vi "GetFileCreationDate.vi"(6 "error in (no error)":errorcluster, 9 "File Path":path) -> (0 "error out":errorcluster, 3 "File Created Date (UTC)":timestamp)   [LabVIEW 2010, in "CAN Log Transfer and Convert.lvlib"]
uses:
  CAN Log Transfer and Convert.lvlib
  kernel32.dll
panel:
  in  "date time rec":T1
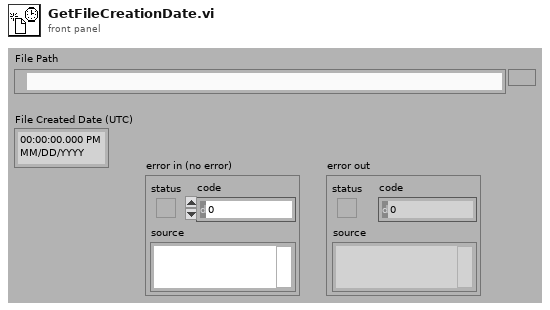
[diagram p1: front panel]
types:
  T1 = cluster{"fractional second":dbl, "second":i32, "minute":i32, "hour":i32, "day of month":i32, "month":i32, "year":i32, "day of week":i32, "day of year":i32, "DST":i32}
  T2 = cluster{"wYear":u16, "wMonth":u16, "wDayOfWeek":u16, "wDay":u16, "wHour":u16, "wMinute":u16, "wSeconds":u16, "wMilliseconds":u16}
  T3 = cluster{"dwFileAttributes":i32, "ftCreationTime":cluster{"dwLowDateTime":i32, "dwHighDateTime":i32}, "ftLastAccessTime":cluster{"dwLowDateTime":i32, "dwHighDateTime":i32}, "ftLastWrittenTime":cluster{"dwLowDateTime":i32, "dwHighDateTime":i32}, "nFileSizeHigh":i32, "nFileSizeLow":i32}
  T4 = cluster{"dwLowDateTime":i32, "dwHighDateTime":i32}
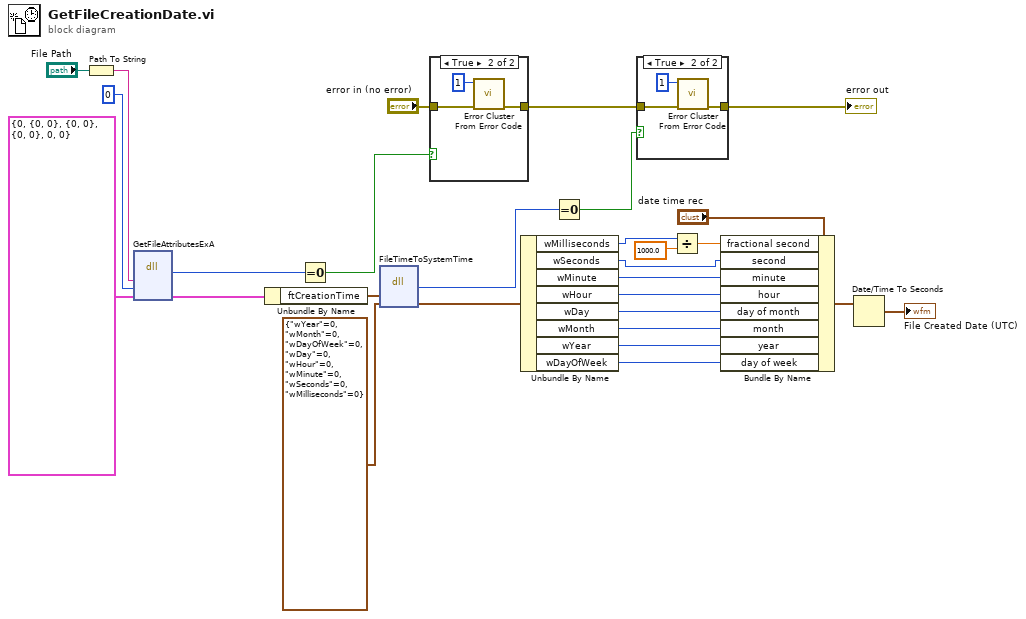
[diagram p0: block diagram]
diagram:
  n1 = Path To String(path="File Path") -> (string=w27:string)
  n2 = dll-call lib="kernel32.dll" fn="GetFileAttributesExA" label="GetFileAttributesEx"("lpFileName"=w27, "fInfoLevelID"=0, "output param"=T3 {"dwFileAttributes"=0, "ftCreationTime"={"dwLowDateTime"=0, "dwHighDateTime"=0}, "ftLastAccessTime"={"dwLowDateTime"=0, "dwHighDateTime"=0}, "ftLastWrittenTime"={"dwLowDateTime"=0, "dwHighDateTime"=0}, "nFileSizeHigh"=0, "nFileSizeLow"=0}) -> (w6:i32, "output param"=w24:T3)  [unwired: 5 in, 2 out]
  n3 = Unbundle By Name(w24) -> ("ftCreationTime"=w23:T4)
  n4 = Equal To 0?(x=w6) -> (x = 0?=w5:bool)
  n5 = dll-call lib="kernel32.dll" fn="FileTimeToSystemTime"("ftCreationTime"=w23, "output param"=T2 {"wYear"=0, "wMonth"=0, "wDayOfWeek"=0, "wDay"=0, "wHour"=0, "wMinute"=0, "wSeconds"=0, "wMilliseconds"=0}) -> (w1:i32, "output param"=w21:T2)  [unwired: 4 in, 2 out]
  n6 = case shown="True" w5 {
    tunnel: "error in (no error)" -> [w29 w32]
    tunnel: [w29 w31] -> w4
    frame False {
    }
    frame True {
      n7 = call <vilib>:"Error Cluster From Error Code.vi"("error in (no error)"=w32, "error code (0)"=1) -> ("error out"=w31:errorcluster)  [unwired: 7 in]
    }
  }
  n8 = Unbundle By Name(w21) -> ("wMilliseconds"=w10:u16, "wSeconds"=w20:u16, "wMinute"=w19:u16, "wHour"=w18:u16, "wDay"=w17:u16, "wMonth"=w16:u16, "wYear"=w15:u16, "wDayOfWeek"=w14:u16)
  n9 = Equal To 0?(x=w1) -> (x = 0?=w2:bool)
  n10 = case shown="True" w2 {
    tunnel: w4 -> [w33 w36]
    tunnel: [w33 w35] -> w3
    frame False {
    }
    frame True {
      n11 = call <vilib>:"Error Cluster From Error Code.vi"("error in (no error)"=w36, "error code (0)"=1) -> ("error out"=w35:errorcluster)  [unwired: 7 in]
    }
  }
  "error out" <- w3
  n12 = Divide(x=w10, y=1000.0) -> (x/y=w9:dbl)
  n13 = Bundle By Name(cluster="date time rec", "fractional second"=w9, "second"=w20, "minute"=w19, "hour"=w18, "day of month"=w17, "month"=w16, "year"=w15, "day of week"=w14) -> (w8:T1)
  n14 = Date/Time To Seconds(2:w8) -> (0:→"File Created Date (UTC)":timestamp)  [unwired: 1 in]
